vi "aft_xmpl_Play Waveform.vi"(11 "sound":waveform(dbl)) -> ()   [LabVIEW 2023]
uses:
  <vilib>/sound2/lvsound2.llb/Sound Data Format.ctl
  <vilib>/sound2/lvsound2.llb/Sampling Mode.ctl
  <vilib>/sound2/lvsound2.llb/Sound Output Write (DBL).vi
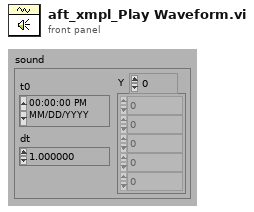
[diagram p1: front panel]
types:
  T1 = typedef "Sampling Mode.ctl" = i32
  T2 = typedef "Sound Data Format.ctl" = cluster{"sample rate (S/s)":dbl, "number of channels":i32, "bits per sample":i32}
  T3 = typedef "Sound Output Task ID.ctl" = u32
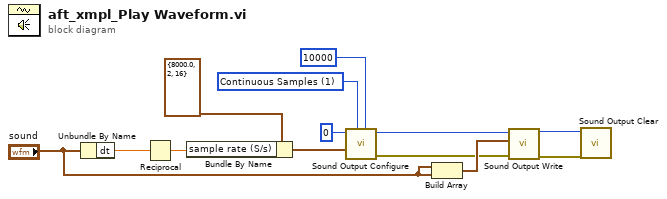
[diagram p0: block diagram]
diagram:
  w10 = T1 1 items=["Finite Samples", "Continuous Samples"] ("sample mode")
  n1 = Unbundle By Name("sound") -> ("dt"=w8:dbl)
  n2 = Reciprocal(x=w8) -> (1/x=w7:dbl)
  n3 = Bundle By Name(cluster=T2 {"sample rate (S/s)"=8000.0, "number of channels"=2, "bits per sample"=16} ("sound format 2"), "sample rate (S/s)"=w7) -> (w11:T2)
  n4 = call <vilib>:"Sound Output Configure.vi"("number of samples/ch"=10000, "sample mode"=w10, "sound format"=w11, "device ID"=u32 0) -> ("error out"=w2:errorcluster, "task ID"=w5:T3)  [unwired: 2 in, 4 out]
  n5 = Build Array("sound", "sound") -> (w4:waveform(dbl)[])
  n6 = call-poly <vilib>:"Sound Output Write.vi"("error in (no error)"=w2, "data"=w4, "task ID"=w5) -> ("error out"=w1:errorcluster, "task ID out"=w6:T3)  [unwired: 1 in, 6 out]
  n7 = call <vilib>:"Sound Output Clear.vi"("error in (no error)"=w1, "task ID"=w6) -> ()  [unwired: 10 out]
